vi "SelectMenu3.vi"(6 "Click Type":T1, 7 "Id":string, 8 "Point":T3, 9 "Item Index":u32, 10 "XRef":refnum<vi>, 11 "State In":T2) -> (0 "Reply":string[](array[string]), 3 "State Out":T2)   [LabVIEW 2018, in "Foreign Key Sort.xnode"]
doc: "This ability VI is called after the user selects an item from a portion of the menu defined during BuildMenu. Click Type is the type of click that led to the building of the menu whose selection is being handled by this VI. ItemIndex is the index of the element in the array used when you specified the popup menu. Id is the id you associated with the item in BuildMenu3. Point is the location where the user clicked to build the menu relative to the top-left corner of the XNode. You can display a dialog in response to a user selection if you wish. Use Reply to inform LabVIEW of any actions it needs to take.\n\nDefault behavior: None.\n\nThis ability provides UI and OS messages are handled.\n\nSee also: BuildMenu3"
uses:
  Foreign Key Sort.xnode
  State.ctl
  <vilib>/XNodeSupport/XNodePoint.ctl
  <vilib>/XNodeSupport/XNodeInt.ctl
  <vilib>/XNodeSupport/XNodeClickTypes.ctl
  <vilib>/XNodeSupport/NI_XNodeSupport.lvlib
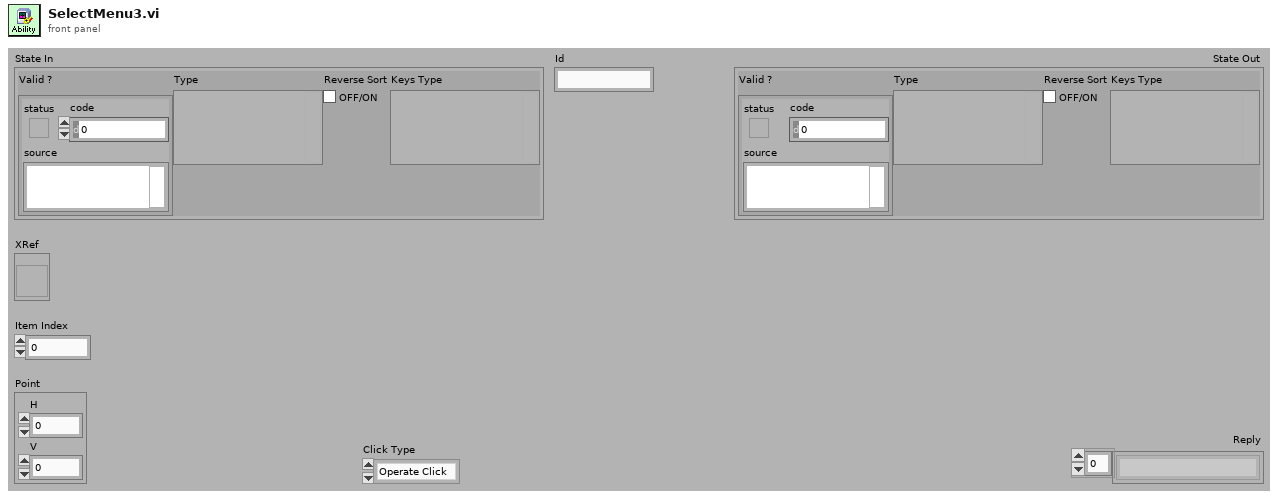
[diagram p1: front panel]
types:
  T1 = typedef "NI_XNodeSupport.lvlib/XNodeClickTypes.ctl" = enum32{"Operate Click", "Popup Click"}
  T2 = typedef "Foreign Key Sort.xnode/State.ctl" = cluster{"Valid ?":errorcluster, "Type":variant, "Reverse Sort":bool, "Keys Type":variant}
  T3 = typedef "NI_XNodeSupport.lvlib/XNodePoint.ctl" = cluster{"H":T4, "V":T4}
  T4 = typedef "NI_XNodeSupport.lvlib/XNodeInt.ctl" = i32
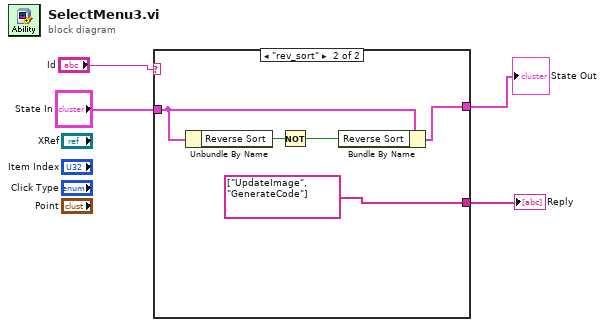
[diagram p0: block diagram]
diagram:
  n1 = case shown="\"rev_sort\"" "Id" {
    tunnel: "State In" -> [w5 w9]
    tunnel: [w5 w7] -> w2
    tunnel: [_ string[] ["UpdateImage", "GenerateCode"] ("Reply")] -> w1
    frame "False", Default {
    }
    frame "rev_sort" {
      n2 = Unbundle By Name(w9) -> ("Reverse Sort"=w10:bool)
      n3 = Not(x=w10) -> (.not. x?=w8:bool)
      n4 = Bundle By Name(cluster=w9, "Reverse Sort"=w8) -> (w7:T2)
    }
  }
  "State Out" <- w2
  "Reply" <- w1
